vi "read data.vi"(8 "error in (no error)":errorcluster, 11 "Device in":T1) -> (0 "error out":errorcluster, 2 "data":string, 3 "Device out":T1)   [LabVIEW 2015]
uses:
  typedefs/device.ctl
panel:
  out "TCP":refnum<k5>
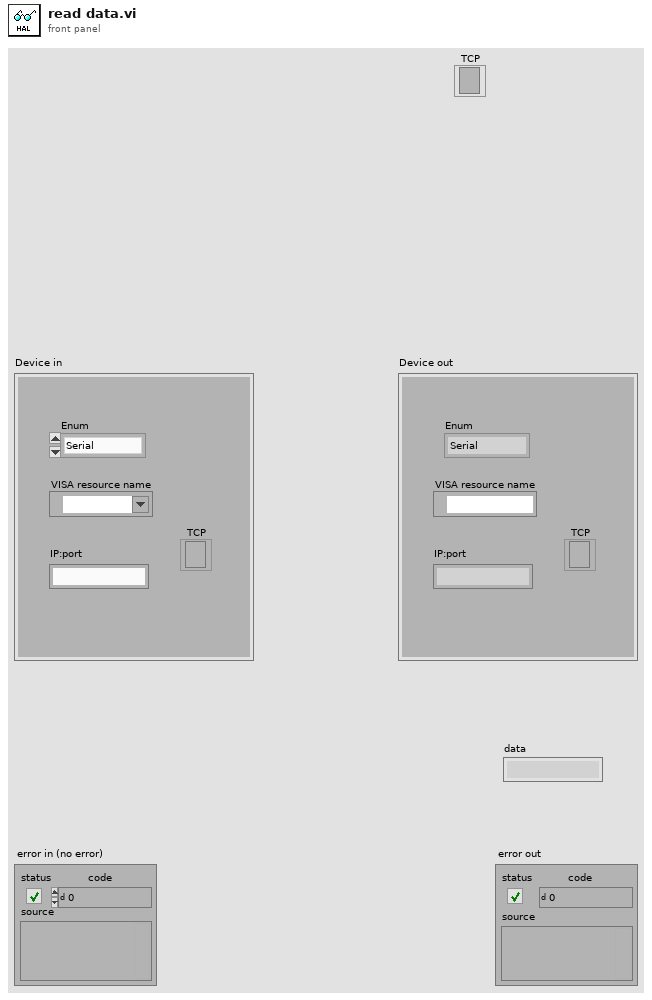
[diagram p1: front panel]
types:
  T1 = typedef "device.ctl" = cluster{"Enum":enum16{"Serial", "TCP/IP", "Mock"}, "IP:port":string, "VISA resource name":refnum<visa-resource-name>, "TCP":refnum<k5>}
  T2 = enum16{"Standard", "Buffered", "CRLF", "Immediate"}
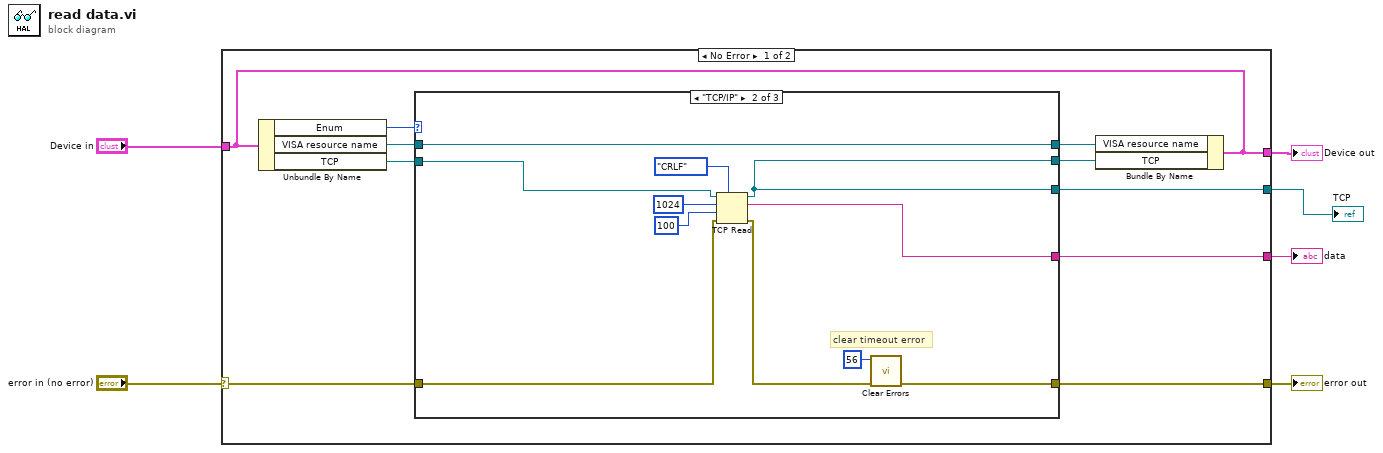
[diagram p0: block diagram]
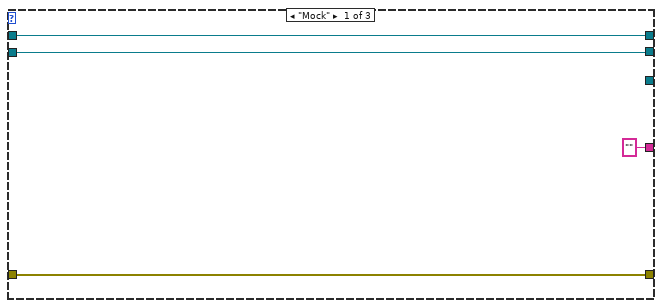
[diagram p2: hidden frame]
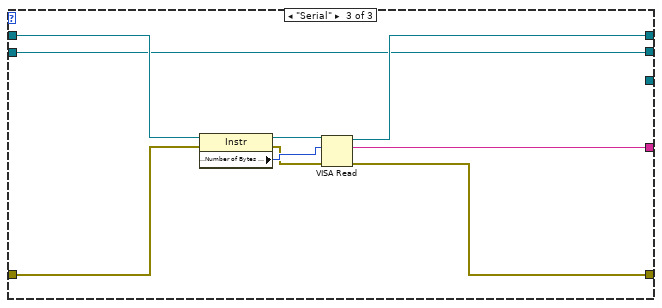
[diagram p3: hidden frame]
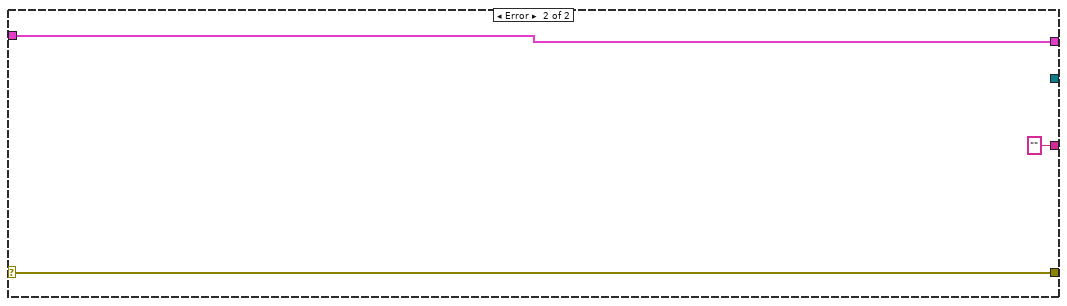
[diagram p4: hidden frame]
diagram:
  n1 = case shown="No Error" "error in (no error)" {
    selector: "error in (no error)" -> [w16 w42]
    tunnel: [w11 w43] -> w5
    tunnel: "Device in" -> [w11 w43]
    tunnel: [w15 w42] -> w3
    tunnel: [w10 "" ("read buffer")] -> w2
    tunnel: [w7 _] -> w1
    frame No Error {
      n2 = Unbundle By Name(w11) -> ("Enum"=w13:enum16{"Serial", "TCP/IP", "Mock"}, "VISA resource name"=w14:refnum<visa-resource-name>, "TCP"=w9:refnum<k5>)
      n3 = case shown="\"TCP/IP\"" w13 {
        tunnel: w14 -> [w20 w31 w37]
        tunnel: w16 -> [w19 w27 w36]
        tunnel: [w19 w23 w33] -> w15
        tunnel: [w20 w31 w35] -> w12
        tunnel: ["" ("read buffer") w26 w34] -> w10
        tunnel: w9 -> [w17 w25 w32]
        tunnel: [w17 w24 w32] -> w8
        tunnel: [_ w24 _] -> w7
        frame "Mock" {
        }
        frame "TCP/IP" {
          # "clear timeout error"
          n4 = TCP Read(connection ID=w25, bytes to read=1024, error in (no error)=w27, 7:T2."CRLF" ("mode (standard)"), 9:100 ("timeout ms (25000)")) -> (connection ID out=w24:refnum<k5>, data out=w26:string, error out=w22:errorcluster)
          n5 = call <vilib>:"Clear Errors.vi"("error in (no error)"=w22, "specific error code to clear (0: all)"=56) -> ("error out"=w23:errorcluster)  [unwired: 4 in, 1 out]
        }
        frame "Serial" {
          n6 = property class="Instr"(reference=w37, error in=w36) -> (reference out=w38:refnum<visa-resource-name>, error out=w39:errorcluster, "Serial Settings:Number of Bytes at Serial Port"=w40:u32)
          n7 = VISA Read(VISA resource name=w38, byte count=w40, error in (no error)=w39) -> (VISA resource name out=w35:refnum<visa-resource-name>, read buffer=w34:string, error out=w33:errorcluster)  [unwired: 1 out]
        }
      }
      n8 = Bundle By Name(cluster=w11, "VISA resource name"=w12, "TCP"=w8) -> ()  [unwired: 1 out]
    }
    frame Error {
    }
  }
  "error out" <- w3
  "Device out" <- w5
  "data" <- w2
  "TCP" <- w1
